vi "Set DataType.vi"(8 "error in":errorcluster, 10 "Value":refnum<class "Value.lvclass">, 11 "DOMAIN in":refnum<class "DOMAIN.lvclass">) -> (0 "error out":errorcluster, 3 "DOMAIN out":refnum<class "DOMAIN.lvclass">)   [LabVIEW 2024, in "Electronic Datasheet.lvlib" / "DOMAIN.lvclass"]
uses:
  DOMAIN.lvclass
  Value/Value.lvclass
  Object Type/Object Type Base.lvclass
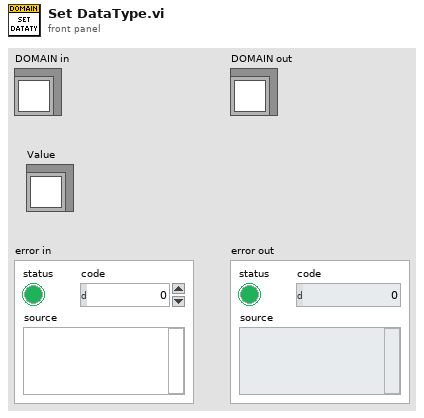
[diagram p1: front panel]
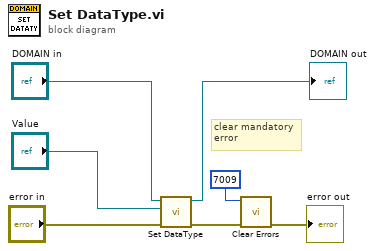
[diagram p0: block diagram]
diagram:
  # "clear mandatory\nerror"
  n1 = call-parent "Set DataType.vi"("error in"="error in", "Value"="Value", "Object Type in"="DOMAIN in") -> ("error out"=w6:errorcluster, "Object Type out"=→"DOMAIN out":refnum<class "DOMAIN.lvclass">)  [unwired: 7 in]
  n2 = call <vilib>:"Clear Errors.vi"("error in (no error)"=w6, "specific error code to clear (0: all)"=7009) -> ("error out"=→"error out":errorcluster)  [unwired: 4 in, 1 out]
